vi "Intan_ADC_Calibrate.vi"(3 "error in":errorcluster, 5 "VISA resource name":refnum<visa-resource-name>="COM1") -> (0 "error out":errorcluster, 1 "Text response":string, 2 "VISA resource name out":refnum<visa-resource-name>)   [LabVIEW 2015]
doc: "Use this VI to perform ADC self-calibration. This should be called AFTER configuring filters (and other registers)."
panel:
  in  "Teensy event char":string="a"
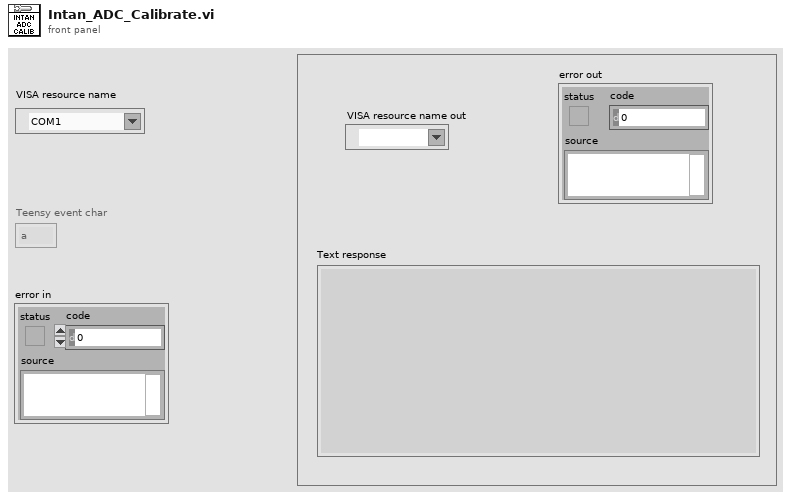
[diagram p1: front panel]
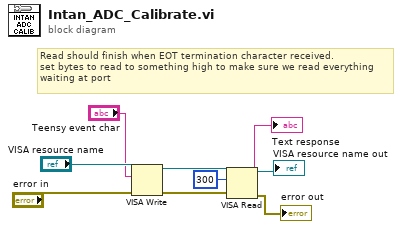
[diagram p0: block diagram]
diagram:
  # "Read should finish when EOT termination character received. \nset bytes to read to something high to make sure we read everything waiting at port"
  n1 = VISA Write(VISA resource name="VISA resource name", write buffer="Teensy event char", error in (no error)="error in") -> (VISA resource name out=w3:refnum<visa-resource-name>, error out=w2:errorcluster)  [unwired: 1 out]
  n2 = VISA Read(VISA resource name=w3, byte count=u32 300, error in (no error)=w2) -> (VISA resource name out=→"VISA resource name out":refnum<visa-resource-name>, read buffer=→"Text response":string, error out=→"error out":errorcluster)  [unwired: 1 out]
